vi "Read Status.vi"(8 "error in (no error)":errorcluster, 11 "SimulationMotor in":refnum<class "SimulationMotor.lvclass">) -> (0 "error out":errorcluster, 2 "Status":T1, 3 "SimulationMotor out":refnum<class "SimulationMotor.lvclass">)   [LabVIEW 2016, in "SimulationMotor.lvclass"]
uses:
  SimulationMotor.lvclass
  motor-drive/Globals/Status--cluster.ctl
  motor-drive/MotorDrive.lvclass
panel:
  in  "Status 2":T1
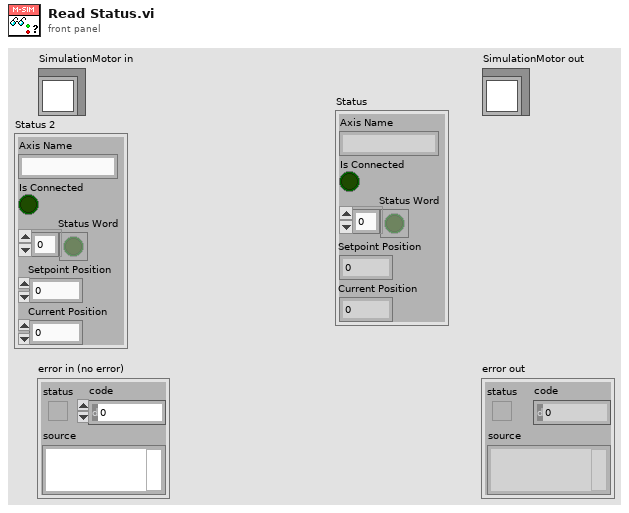
[diagram p1: front panel]
types:
  T1 = typedef "MotorDrive.lvclass/Status--cluster.ctl" = cluster{"Axis Name":string, "Is Connected":bool, "Status Word":bool[], "Setpoint Position":dbl, "Current Position":dbl}
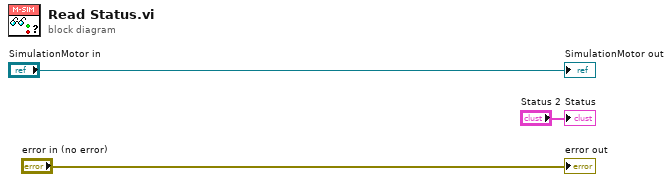
[diagram p0: block diagram]
diagram:
  "error out" <- "error in (no error)"
  "SimulationMotor out" <- "SimulationMotor in"
  "Status" <- "Status 2"
